vi "Repack Package.vi"(4 "Delete Directory to repack (TRUE)?":bool=TRUE, 6 "Overwrite Target Package File (True)?":bool=TRUE, 7 "Package File (\"\": use name of directory to repack)":path, 8 "error in (no error)":errorcluster, 11 "Directory to repack":path) -> (0 "error out":errorcluster)   [LabVIEW 2020]
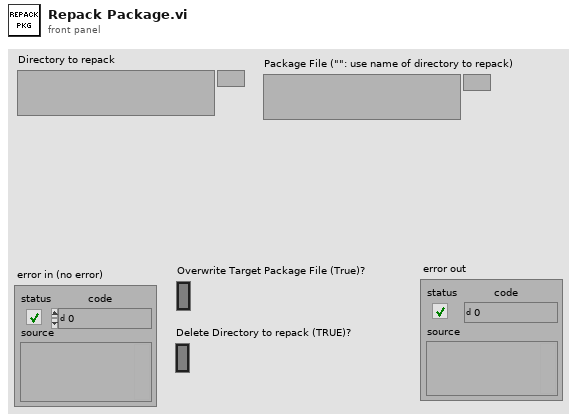
[diagram p1: front panel]
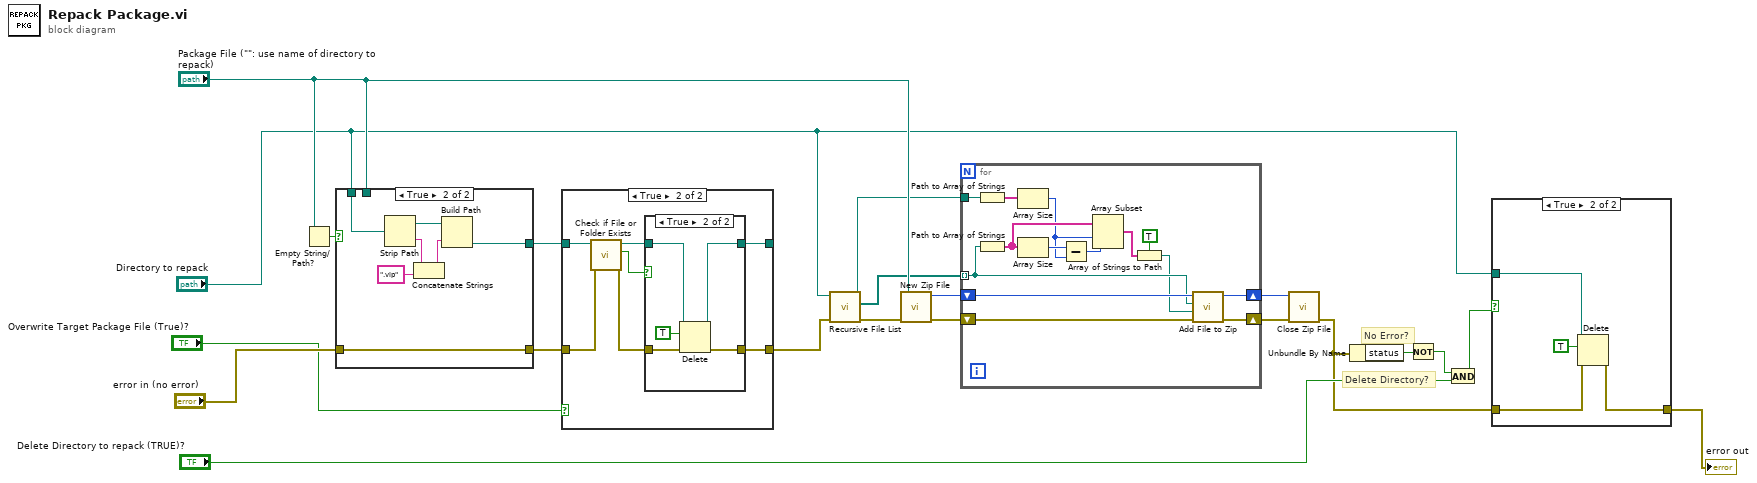
[diagram p0: block diagram]
diagram:
  # "Delete Directory?"
  # "No Error?"
  n1 = Empty String/Path?(string/path="Package File (\"\": use name of directory to repack)") -> (empty?=w21:bool)
  n2 = case shown="True" w21 {
    tunnel: "Package File (\"\": use name of directory to repack)" -> [w22 _]
    tunnel: "error in (no error)" -> [w23 w25]
    tunnel: [w23 w25] -> w19
    tunnel: [w22 w29] -> w18
    tunnel: "Directory to repack" -> [_ w24]
    frame False {
    }
    frame True {
      n3 = Strip Path(path=w24) -> (stripped path=w30:path, name=w28:string)
      n4 = Concatenate Strings(w28, ".vip" ("string")) -> (w27:string)
      n5 = Build Path(base path=w30, name or relative path=w27) -> (appended path=w29:path)
    }
  }
  n6 = case shown="True" "Overwrite Target Package File (True)?" {
    tunnel: w19 -> [w31 w39]
    tunnel: w18 -> [w32 w38]
    tunnel: [w32 w34] -> _
    tunnel: [w31 w33] -> w16
    frame False {
    }
    frame True {
      n7 = call <vilib>:"Check if File or Folder Exists.vi"("error in (no error)"=w39, "path"=w38) -> ("error out"=w36:errorcluster, "file or folder exists?"=w37:bool, "dup path"=w35:path)  [unwired: 7 in]
      n8 = case shown="True" w37 {
        tunnel: w36 -> [w41 w46]
        tunnel: w35 -> [w40 w44]
        tunnel: [w40 w43] -> w34
        tunnel: [w41 w42] -> w33
        frame False {
        }
        frame True {
          n9 = Delete(path (use dialog)=w44, entire hierarchy (F)=TRUE, error in=w46) -> (deleted path=w43:path, error out=w42:errorcluster)  [unwired: 2 in, 1 out]
        }
      }
    }
  }
  n10 = call <vilib>:"Recursive File List.vi"("error in (no error)"=w16, "Folder Path"="Directory to repack") -> ("error out"=w14:errorcluster, "All Files in Dir"=w13:path[], "dup Folder Path"=w8:path)  [unwired: 5 in, 2 out]
  n11 = call <vilib>:"New Zip File.vi"("error in (no error)"=w14, "target"="Package File (\"\": use name of directory to repack)") -> ("error out"=w12:errorcluster, "zip file out"=w11:i64)  [unwired: 3 in, 1 out]
  n12 = for {
    tunnel: w13 -> [w55] mode=indexing
    shift-right: [w58] -> w10
    shift-left: w12 -> [w60]
    shift-right: [w57] -> w9
    shift-left: w11 -> [w59]
    tunnel: w8 -> [w56]
    n13 = Path to Array of Strings(0:w56) -> (2:w54:string[])  [unwired: 1 out]
    n14 = Path to Array of Strings(0:w55) -> (2:w53:string[])  [unwired: 1 out]
    n15 = Array Size(array=w54) -> (size(s)=w51:i32)
    n16 = Array Size(array=w53) -> (size(s)=w52:i32)
    n17 = Subtract(x=w52, y=w51) -> (x-y=w50:i32)
    n18 = Array Subset(array=w53, index=w51, length=w50) -> (w49:string[])
    n19 = Array of Strings to Path(0:w49, 1:TRUE ("relative")) -> (2:w47:path)
    n20 = call <vilib>:"Add File to Zip.vi"("error in (no error)"=w60, "destination path in zip"=w47, "source file path"=w55, "zip file in"=w59) -> ("error out"=w58:errorcluster, "zip file out"=w57:i64)  [unwired: 6 in]
  }
  n21 = call <vilib>:"Close Zip File.vi"("error in (no error)"=w10, "zip file in"=w9) -> ("error out"=w3:errorcluster)  [unwired: 5 in]
  n22 = Unbundle By Name(w3) -> ("status"=w7:bool)
  n23 = Not(x=w7) -> (.not. x?=w6:bool)
  n24 = And(x=w6, y="Delete Directory to repack (TRUE)?") -> (x .and. y?=w4:bool)
  n25 = case shown="True" w4 {
    tunnel: w3 -> [w61 w64]
    tunnel: "Directory to repack" -> [_ w63]
    tunnel: [w61 w62] -> w2
    frame False {
    }
    frame True {
      n26 = Delete(path (use dialog)=w63, entire hierarchy (F)=TRUE, error in=w64) -> (error out=w62:errorcluster)  [unwired: 2 in, 2 out]
    }
  }
  "error out" <- w2
